vi "Mcp2210 Get Gpio Pin Dir.vi"(8 "error in (no error)":errorcluster, 10 "GPIO Direction":bool[](array[boolean]), 11 "handle":i32) -> (0 "error out":errorcluster, 3 "handle out":i32)   [LabVIEW 2015, in "mcp2210.lvlib"]
doc: "Provides the current GPIO pin direction. The values are valid only for the pins\npreviously configured as GPIOs.\nParameters:\nInputs:\n- void *handle - The pointer to the device handle. Cannot be NULL.\nOutputs:\n- unsigned int *pgpioDir - GPIO pin direction, if successful call. In case of error the value\nis not changed.\nCannot be NULL pointer.\nReturns:\n- 0 for success: E_SUCCESS\n- negative error code: E_ERR_NULL, E_ERR_INVALID_HANDLE_VALUE\nE_ERR_UNKOWN_ERROR, E_ERR_INVALID_PARAMETER\nE_ERR_HID_TIMEOUT, E_ERR_HID_RW_FILEIO\nE_ERR_CMD_ECHO, E_ERR_CMD_FAILED\n\nMCP2210_DLL_UM_API int __stdcall Mcp2210_GetGpioPinDir(void *handle, unsigned int *pgpioDir);"
uses:
  <userlib>/mcp2210/mcp2210.lvlib
  <userlib>/mcp2210/mcp2210_dll_um_x86.dll
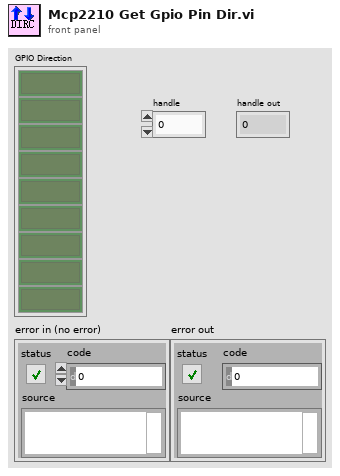
[diagram p1: front panel]
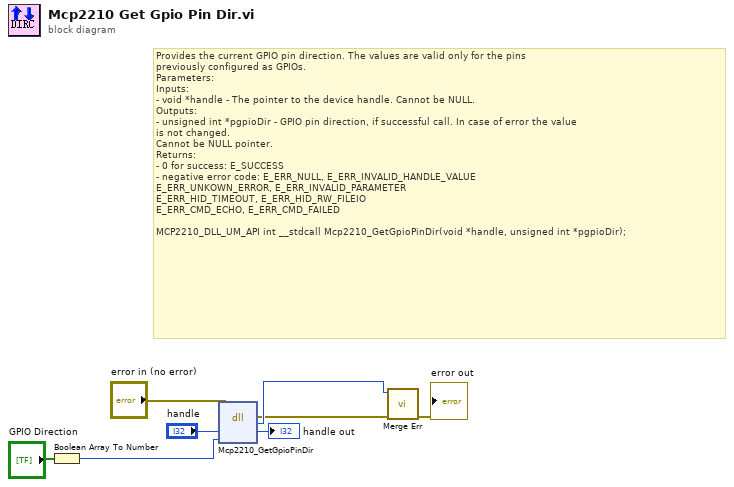
[diagram p0: block diagram]
diagram:
  # "Provides the current GPIO pin direction. The values are valid only for the pins\npreviously configured as GPIOs.\nParameters:\nInputs:\n- void *handle - The pointer to the device handle. Cannot be NULL.\nOutputs:\n- unsigned int *pgpioDir - GPIO pin direction, if successful call. In case of error the value\nis not changed.\nCannot be NULL pointer.\nReturns:\n- 0 for success: E_SUCCESS\n- negative error code: E_ERR_NULL, E_ERR_INVALID_HANDLE_VALUE\nE_ERR_UNKOWN_ERROR, E_ERR_INVALID_PARAMETER\nE_ERR_HID_TIMEOUT, E_ERR_HID_RW_FILEIO\nE_ERR_CMD_ECHO, E_ERR_CMD_FAILED\n\nMCP2210_DLL_UM_API int __stdcall Mcp2210_GetGpioPinDir(void *handle, unsigned int *pgpioDir);"
  n1 = Boolean Array To Number(Boolean array="GPIO Direction") -> (number=w1:u32)
  n2 = dll-call lib="D:/LabVIEW 2015/user.lib/mcp2210/mcp2210_dll_um_x86.*" fn="Mcp2210_GetGpioPinDir"(error in="error in (no error)", "handle"="handle", "pgpioDir"=w1) -> (error out=w5:errorcluster, "return type"=w6:i32, "handle"=→"handle out":i32)  [unwired: 3 in, 1 out]
  n3 = call <userlib>:"Merge Err.vi"("error in (no error)"=w5, "return type"=w6) -> ("error out"=→"error out":errorcluster)  [unwired: 9 in]
